vi "Server.vi"() -> ()   [LabVIEW 2020]
panel:
  in  "stop":bool
  out "error out":errorcluster
  in  "data in":string
  # "Server"
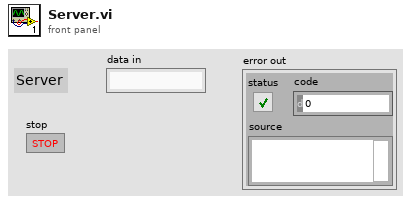
[diagram p1: front panel]
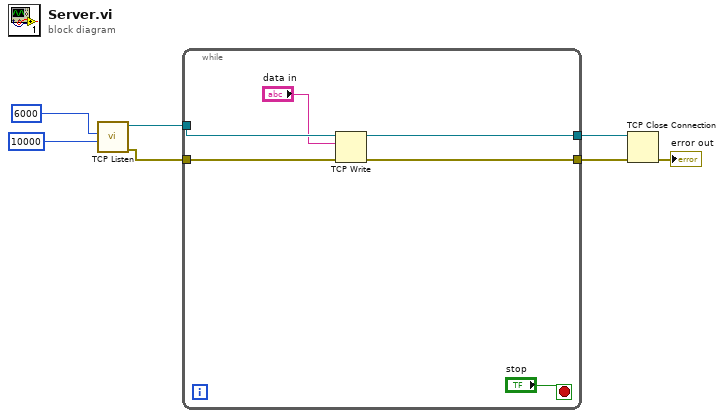
[diagram p0: block diagram]
diagram:
  n1 = call <vilib>:"TCP Listen.vi"("timeout ms (wait forever: -1)"=10000, "port"=u16 6000) -> ("error out"=w5:errorcluster, "connection ID"=w7:refnum<k5>)  [unwired: 5 in, 3 out]
  n2 = while {
    tunnel: w7 -> [w13]
    tunnel: [w12] -> w6
    tunnel: w5 -> [w11]
    tunnel: [w10] -> w4
    stop <- "stop" stop-if-true
    n3 = TCP Write(connection ID=w13, data in="data in", error in (no error)=w11) -> (connection ID out=w12:refnum<k5>, error out=w10:errorcluster)  [unwired: 1 in, 1 out]
  }
  n4 = TCP Close Connection(connection ID=w6, error in (no error)=w4) -> (error out=→"error out":errorcluster)  [unwired: 1 in, 1 out]
